vi "Set SPI Sample Rate.vi"(8 "error in (no error)":errorcluster, 10 "Sample Rate (S/s)":u32, 11 "Item Ref in":T1 format="%.0x") -> (0 "error out":errorcluster, 3 "Item Ref out":T1 format="%.0x")   [LabVIEW 2014, in "SLSC configuration System Explorer.lvlib"]
uses:
  SLSC configuration System Explorer.lvlib
  <vilib>/NI Veristand/Custom Device API/Custom Device Item Ref.ctl
  Shared/Constants.vi
  <vilib>/NI Veristand/Custom Device API/Set Item Property (U32).vi
  <vilib>/NI Veristand/Custom Device API/Custom Device API.lvlib
  Shared/SLSC configuration Shared.lvlib
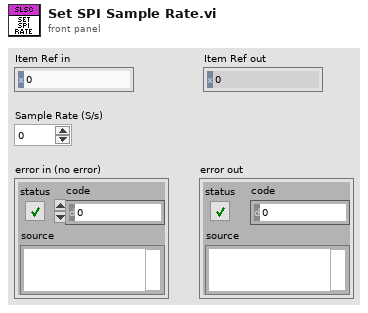
[diagram p1: front panel]
types:
  T1 = typedef "Custom Device API.lvlib/Custom Device Item Ref.ctl" = u64
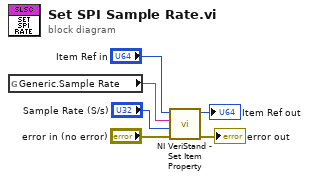
[diagram p0: block diagram]
diagram:
  n1 = global read "Constants.vi" "Generic.Sample Rate"() -> (w5:string)
  n2 = call-poly <vilib>:"NI VeriStand - Set Item Property.vi"("error in (no error)"="error in (no error)", "Value"="Sample Rate (S/s)", "Property Name"=w5, "Item Ref in"="Item Ref in") -> ("error out"=→"error out":errorcluster, "Item Ref out"=→"Item Ref out":T1)  [unwired: 5 in, 1 out]
